vi "Calibration Interpolation (Set).vi"(6 "ISOBUS address":T4=-1 caption="ISOBUS address (-1)", 8 "error in":errorcluster, 10 "Calibration Interpolation":T3, 11 "Mercury Reference In":T5) -> (0 "error out":errorcluster, 2 "Response":T1, 3 "Mercury Reference Out":T5, 4 "Valid?":T2)   [LabVIEW 2014, in "Mercury iXX.lvlib" / "Pressure.lvlib"]
doc: "Set the current interpolation method of the selected pressure device."
uses:
  Pressure.lvlib
  Controls/Mercury Reference.ctl
  Controls/Comms Transport Layer.ctl
  Private/Controls/Query Dynamic Reference.ctl
  Controls/ISOBus Address.ctl
  Controls/Calibration Interpolation.ctl
  Controls/Is Valid LED.ctl
  Controls/Response String.ctl
  Private/Controls/Command Verbs.ctl
  Mercury iXX.lvlib
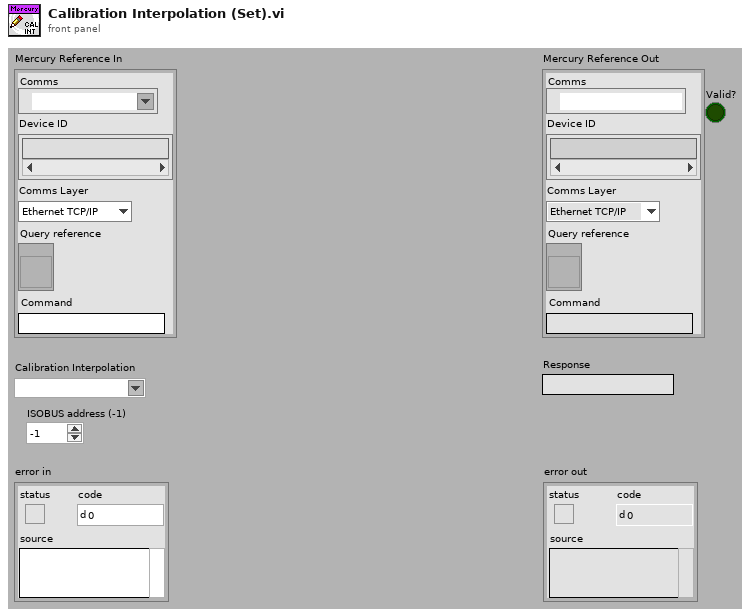
[diagram p1: front panel]
types:
  T1 = typedef "Mercury iXX.lvlib/Response String.ctl" = string
  T2 = typedef "Mercury iXX.lvlib/Is Valid LED.ctl" = bool
  T3 = typedef "Mercury iXX.lvlib/Pressure.lvlib/Calibration Interpolation.ctl" = string
  T4 = typedef "Mercury iXX.lvlib/ISOBus Address.ctl" = i32
  T5 = typedef "Mercury iXX.lvlib/Mercury Reference.ctl" = cluster{"Comms":refnum<visa-resource-name>, "Device ID":string[], "Comms Layer":T6, "Command":string, "Query reference":T7}
  T6 = typedef "Mercury iXX.lvlib/Comms Transport Layer.ctl" = enum16{"Ethernet TCP/IP", "USB", "ISOBus - RS-232", "GPIB"}
  T7 = typedef "Mercury iXX.lvlib/Query Dynamic Reference.ctl" = refnum<vi>
  T8 = typedef "Mercury iXX.lvlib/Command Verbs.ctl" = string
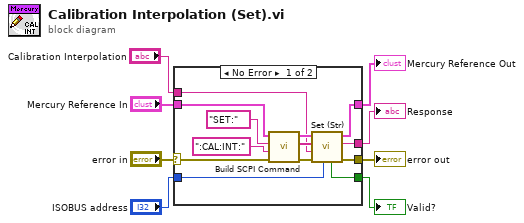
[diagram p0: block diagram]
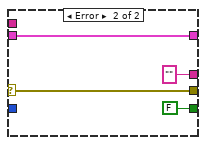
[diagram p2: hidden frame]
diagram:
  n1 = case shown="No Error" "error in" {
    selector: "error in" -> [w9 w25]
    tunnel: "Mercury Reference In" -> [w16 w24]
    tunnel: "Calibration Interpolation" -> [w15 _]
    tunnel: [w14 w24] -> w6
    tunnel: [w13 T1 "" ("Response")] -> w5
    tunnel: [w12 T2 FALSE ("Valid?")] -> w4
    tunnel: [w11 w25] -> w3
    tunnel: "ISOBUS address" -> [w10 _]
    frame No Error {
      n2 = call "Build SCPI Command.vi"("error in"=w9, "Noun(s)"=":CAL:INT:" ("Command"), "Verb"=T8 "SET:", "Mercury Reference In"=w16) -> ("error out"=w18:errorcluster, "SCPI Message(s)"=w19:string[], "Mercury Reference Out"=w20:T5)  [unwired: 5 out]
      n3 = call "Set (Str).vi"("ISOBUS address"=w10, "error in"=w18, "Command Value (Str)"=w15, "SCPI Message(s)"=w19, "Mercury Reference In"=w20) -> ("error out"=w11:errorcluster, "Response"=w13:T1, "Mercury Reference Out"=w14:T5, "Valid?"=w12:T2)  [unwired: 3 out]
    }
    frame Error {
    }
  }
  "Mercury Reference Out" <- w6
  "error out" <- w3
  "Valid?" <- w4
  "Response" <- w5
